vi "Copy Existing Scaffolds from Negentropic.vi"(8 "error in (no error)":errorcluster) -> (0 "error out":errorcluster)   [LabVIEW 2020]
uses:
  Negentropic IDE/Negentropic IDE.lvlib
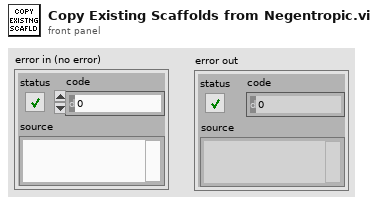
[diagram p1: front panel]
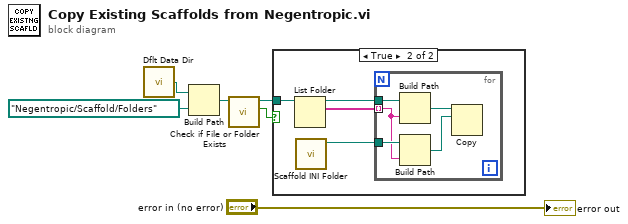
[diagram p0: block diagram]
diagram:
  n1 = call <vilib>:"Dflt Data Dir.vi"() -> ("App:Default Data Directory"=w6:path)
  n2 = Build Path(base path=w6, name or relative path=path "Negentropic/Scaffold/Folders") -> (appended path=w4:path)
  n3 = call <vilib>:"Check if File or Folder Exists.vi"("path"=w4) -> ("file or folder exists?"=w3:bool, "dup path"=w2:path)  [unwired: 8 in, 1 out]
  n4 = case shown="True" w3 {
    tunnel: w2 -> [_ w10]
    frame False {
    }
    frame True {
      n5 = List Folder(path=w10) -> (path out=w7:path, filenames=w8:string[])  [unwired: 3 in, 2 out]
      n6 = call "Scaffold INI Folder.vi"() -> ("Scaffold INI Folder"=w9:path)  [unwired: 10 in, 1 out]
      n7 = for {
        tunnel: w9 -> [w14]
        tunnel: w8 -> [w13] mode=indexing
        tunnel: w7 -> [w15]
        n8 = Build Path(base path=w15, name or relative path=w13) -> (appended path=w12:path)
        n9 = Build Path(base path=w14, name or relative path=w13) -> (appended path=w11:path)
        n10 = Copy(10:w11, 11:w12) -> ()  [unwired: 3 in, 3 out]
      }
    }
  }
  "error out" <- "error in (no error)"
